vi "WaveformCompChange.vi"(1 "component":dbl[](array[numeric]), 2 "input waveform":waveform(dbl)) -> (0 "output waveform":waveform(dbl))   [LabVIEW 2019]
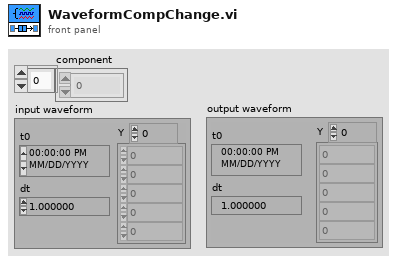
[diagram p1: front panel]
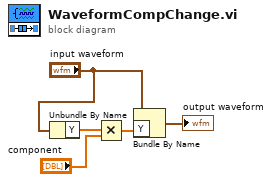
[diagram p0: block diagram]
diagram:
  n1 = Unbundle By Name("input waveform") -> ("Y"=w5:dbl[])
  n2 = Multiply(x=w5, y="component") -> (x*y=w4:dbl[])
  n3 = Bundle By Name(cluster="input waveform", "Y"=w4) -> (→"output waveform":waveform(dbl))
